vi "Draw.vi"(7 "menu in":refnum<class "menu.lvclass">, 8 "error in (no error)":errorcluster, 11 "separator item in":refnum<class "separator item.lvclass">) -> (0 "error out":errorcluster, 3 "separator item out":refnum<class "separator item.lvclass">)   [LabVIEW 2009, in "separator item.lvclass"]
uses:
  separator item.lvclass
  Menu/menu.lvclass
  separator item.lvclass/separator item.ctl
  Menu Item/menu item.lvclass
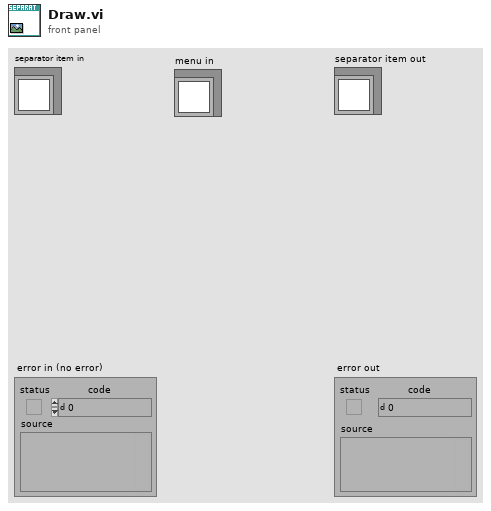
[diagram p1: front panel]
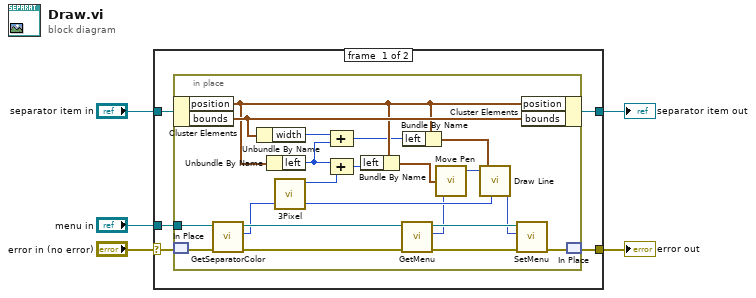
[diagram p0: block diagram]
diagram:
  n1 = case shown="No Error" "error in (no error)" {
    selector: "error in (no error)" -> [w10 w32]
    tunnel: [w9 w32] -> w4
    tunnel: "separator item in" -> [w8 w31]
    tunnel: [w7 w31] -> w2
    tunnel: "menu in" -> [w6 _]
    frame #0 {
      n2 = in-place {
        in-place-border: w6 -> [w30]
        n3 = in-place-cluster #1(w8) -> ("position"=w14:cluster{"left":u32, "top":u32}, "bounds"=w17:cluster{"width":u32, "height":u32})
        n4 = in-place-match #2(w10) -> (w22:errorcluster)
        n5 = call "GetSeparatorColor.vi"("error in (no error)"=w22, "menu in"=w30) -> ("error out"=w23:errorcluster, "separator color"=w26:u32, "menu out"=w29:refnum<class "menu.lvclass">)  [unwired: 7 in]
        n6 = Unbundle By Name(w17) -> ("width"=w16:u32)
        n7 = Unbundle By Name(w14) -> ("left"=w15:u32)
        n8 = call "3Pixel.vi"() -> ("3 pixel"=w11:u32)  [unwired: 11 in]
        n9 = Compound Arithmetic op=ADD(w16, w15) -> (w13:u32)
        n10 = Compound Arithmetic op=ADD(w15, w11) -> (w18:u32)
        n11 = Bundle By Name(cluster=w14, "left"=w18) -> (w19:cluster{"left":u32, "top":u32})
        n12 = call "GetMenu.vi"("error in (no error)"=w23, "menu in"=w29) -> ("error out"=w24:errorcluster, "menu"=w21:picture, "menu out"=w28:refnum<class "menu.lvclass">)  [unwired: 7 in]
        n13 = Bundle By Name(cluster=w14, "left"=w13) -> (w12:cluster{"left":u32, "top":u32})
        n14 = call <vilib>:"Move Pen.vi"("new position"=w19, "picture"=w21) -> ("new picture"=w27:picture)  [unwired: 3 in]
        n15 = call <vilib>:"Draw Line.vi"("picture"=w27, "end point"=w12, "color(black)"=w26) -> ("new picture"=w20:picture)  [unwired: 6 in]
        n16 = call "SetMenu.vi"("error in (no error)"=w24, "menu"=w20, "menu in"=w28) -> ("error out"=w25:errorcluster)  [unwired: 7 in, 1 out]
        n17 = in-place-cluster #1("position"=w14, "bounds"=w17) -> (w7:refnum<class "separator item.lvclass">)
        n18 = in-place-match #2(w25) -> (w9:errorcluster)
      }
    }
    frame #1 {
    }
  }
  "separator item out" <- w2
  "error out" <- w4
